vi "GT Set Watch.vi"(8 "error in (no error)":errorcluster caption="错误输入（无错误）", 10 "pWatch":T1, 11 "cardNum":i16) -> (0 "error out":errorcluster caption="错误输出", 2 "pWatch out":T1, 3 "function return":i16)   [LabVIEW 2020, in "gts1.lvlib"]
doc: "GT_API GT_SetWatch(short cardNum,TWatch *pWatch);"
uses:
  gts1.lvlib
  dll/32bit/multi_card/gts.dll
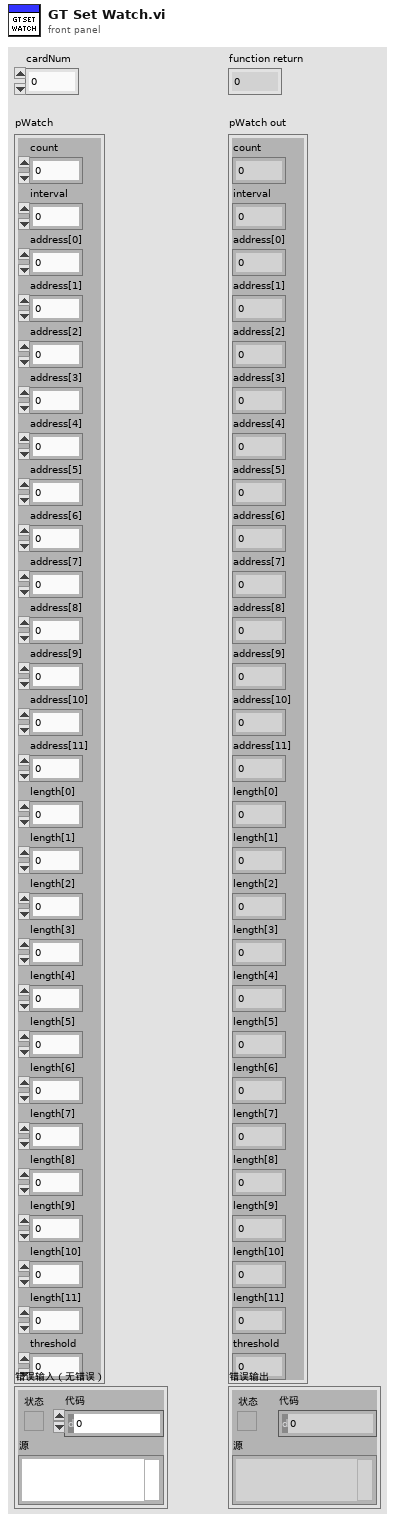
[diagram p1: front panel]
types:
  T1 = cluster{"count":i16, "interval":i16, "address[0]":u32, "address[1]":u32, "address[2]":u32, "address[3]":u32, "address[4]":u32, "address[5]":u32, "address[6]":u32, "address[7]":u32, "address[8]":u32, "address[9]":u32, "address[10]":u32, "address[11]":u32, "length[0]":i16, "length[1]":i16, "length[2]":i16, "length[3]":i16, "length[4]":i16, "length[5]":i16, "length[6]":i16, "length[7]":i16, "length[8]":i16, "length[9]":i16, "length[10]":i16, "length[11]":i16, "threshold":u32}
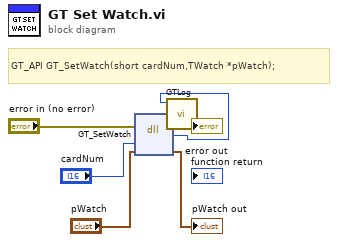
[diagram p0: block diagram]
diagram:
  # "GT_API GT_SetWatch(short cardNum,TWatch *pWatch);"
  n1 = dll-call lib="C:/1228/dll/32bit/multi_card/gts.dll" fn="GT_SetWatch"(error in="error in (no error)", "cardNum"="cardNum", "pWatch"="pWatch") -> (error out=w3:errorcluster, w1:i16, "pWatch"=→"pWatch out":T1)  [unwired: 3 in, 1 out]
  n2 = call "GTLog.vi"("error in (no error)"=w3, "Numeric"=w1) -> ("error out"=→"error out":errorcluster)  [unwired: 9 in]
